vi "Get_Phase_Shift.vi"(1 "Data QY":string, 2 "Data QX":string) -> (0 "Numeric":dbl)   [LabVIEW 2010]
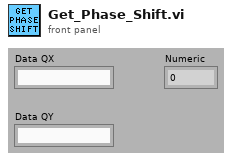
[diagram p1: front panel]
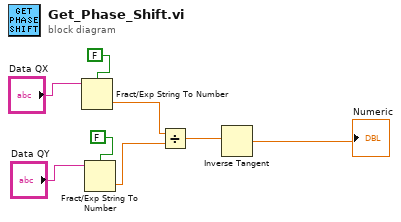
[diagram p0: block diagram]
diagram:
  n1 = Fract/Exp String To Number(use system decimal point (T)=FALSE, string="Data QX") -> (number=w3:dbl)  [unwired: 2 in, 1 out]
  n2 = Fract/Exp String To Number(use system decimal point (T)=FALSE, string="Data QY") -> (number=w4:dbl)  [unwired: 2 in, 1 out]
  n3 = Divide(x=w3, y=w4) -> (x/y=w2:dbl)
  n4 = Inverse Tangent(1:w2) -> (0:→"Numeric":dbl)
